vi "RegisterActionEvent.vi"(8 "error in (no error)":errorcluster, 10 "Action":string, 11 "CONTROLLER in":refnum<class "CONTROLLER.lvclass">) -> (0 "error out":errorcluster, 3 "CONTROLLER out":refnum<class "CONTROLLER.lvclass">)   [LabVIEW 2013, in "CONTROLLER.lvclass"]
uses:
  CONTROLLER.lvclass
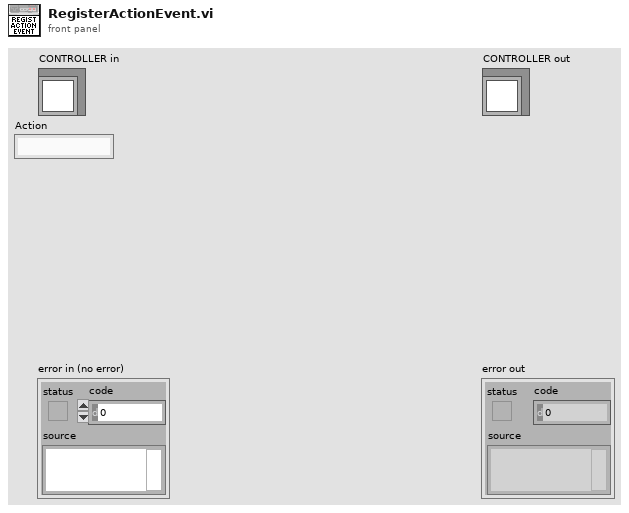
[diagram p1: front panel]
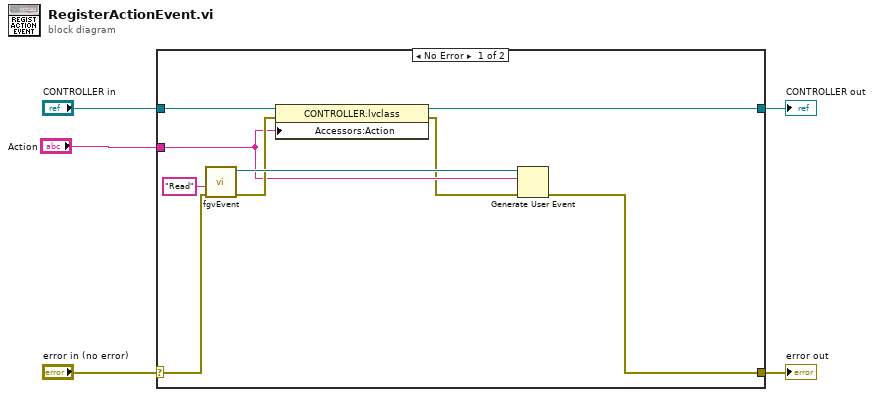
[diagram p0: block diagram]
diagram:
  n1 = case shown="No Error" "error in (no error)" {
    selector: "error in (no error)" -> [w9 w16]
    tunnel: [w13 w16] -> w4
    tunnel: [w10 w15] -> w2
    tunnel: "CONTROLLER in" -> [w11 w15]
    tunnel: "Action" -> [w7 _]
    frame No Error {
      n2 = call "fgvEvent.vi"("error in (no error)"=w9, "Cmd"="Read") -> ("error out"=w8:errorcluster, "eventData Out"=w14:refnum<user-event>)  [unwired: 7 in, 1 out]
      n3 = property class="CONTROLLER.lvclass"(reference=w11, error in=w8, "Accessors:Action"=w7) -> (reference out=w10:refnum<class "CONTROLLER.lvclass">, error out=w6:errorcluster)
      n4 = Generate User Event(user event=w14, event data cluster=w7, error in=w6) -> (error out=w13:errorcluster)  [unwired: 1 in, 1 out]
    }
    frame Error {
    }
  }
  "error out" <- w4
  "CONTROLLER out" <- w2
